vi "real_cell_number.vi"(0 "1st":dbl, 1 "2nd":dbl, 2 "3rd":dbl, 3 "4th":dbl, 4 "current loop (cell)":i32) -> (5 "real cell number":dbl)   [LabVIEW 2016]
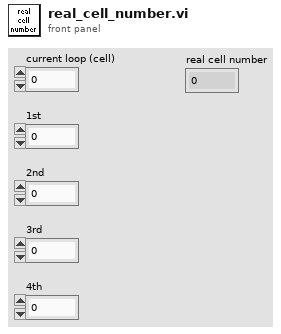
[diagram p1: front panel]
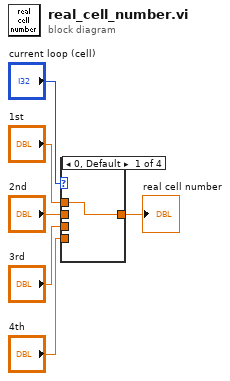
[diagram p0: block diagram]
diagram:
  n1 = case shown="0, Default" "current loop (cell)" {
    tunnel: [w7 w8 w9 w10] -> w6
    tunnel: "1st" -> [w7 _ _ _]
    tunnel: "2nd" -> [_ w8 _ _]
    tunnel: "3rd" -> [_ _ w9 _]
    tunnel: "4th" -> [_ _ _ w10]
    frame 0, Default {
    }
    frame 1 {
    }
    frame 2 {
    }
    frame 3 {
    }
  }
  "real cell number" <- w6
